vi "PSCOMMON_Toolbar Comond.vi"(7 "Pause？":bool, 8 "error in":errorcluster, 11 "Command":enum16{"Config", "Run", "Pause", "Stop", "Save"}(ring)) -> (0 "error out":errorcluster)   [LabVIEW 2016]
uses:
  X-Acquisition/DAQ Actor/API/PSDAQEG_Commoand Type.ctl
  Controls/Save Mode.ctl
  Ctrls/GlobeVaribles.vi
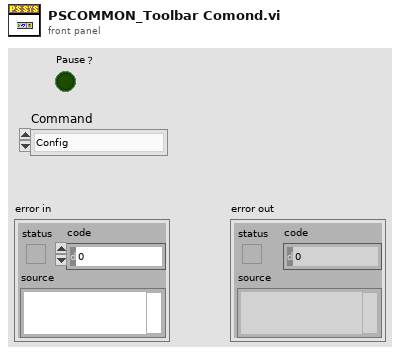
[diagram p1: front panel]
types:
  T1 = typedef "PSDAQEG_Commoand Type.ctl" = enum16{"Config", "Run", "Pause", "Stop", "Save"}
  T2 = enum16{"Run", "Pause", "Stop", "DAQ Chl", "Save", "Update Data", "Symbol Path", "DAQ DATA Queues", "None"}
  T3 = enum16{"Run", "Pause", "Stop", "DAQ Chl", "Save", "Update Data"}
  T4 = enum16{"open", "open or create", "create or replace", "create", "open (read-only)"}
  T5 = typedef "Global para Config.ctl" = cluster{"Timing":cluster{"SampleRate":i32}, "SavePara":cluster{"FlowDiskMode":T6, "SelectMode":T7, "FolderPath":path, "Filename":string, "FileNote":string, "AutoInterval":i32, "Template":path}, "ConfigDS Path*":path, "Tdms Ref*":refnum<k34>}
  T6 = typedef "File Save Mode.ctl" = i32
  T7 = typedef "Select Point Mode.ctl" = i32
  T8 = typedef "Save Mode.ctl" = i32
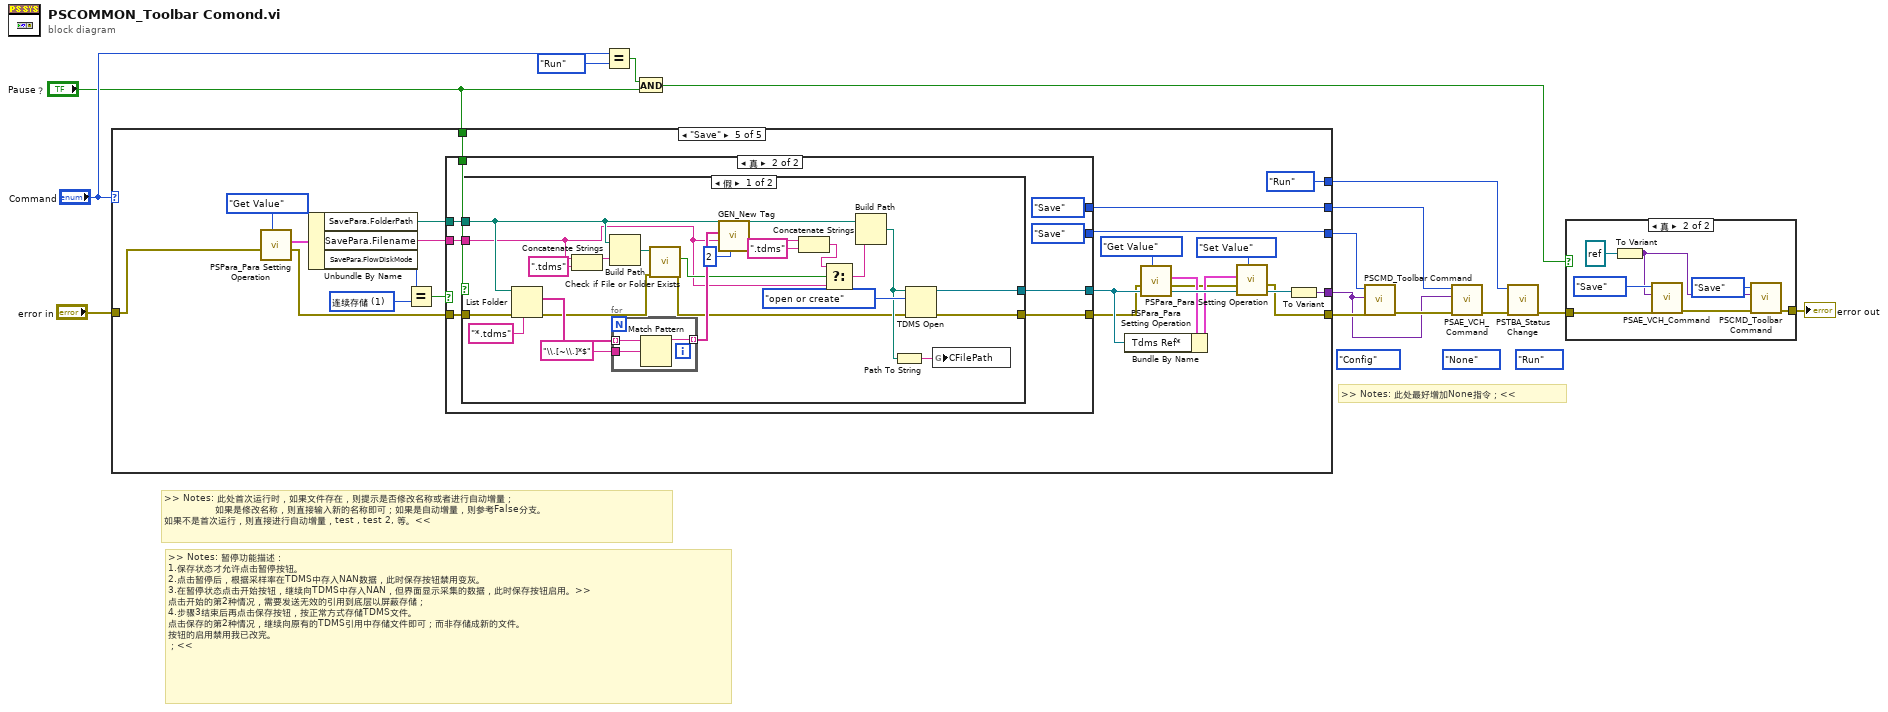
[diagram p0: block diagram]
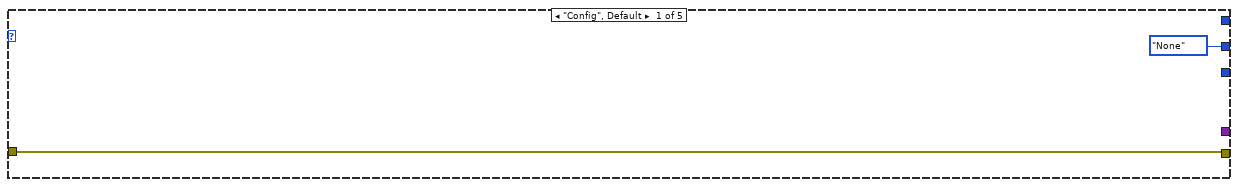
[diagram p3: hidden frame]
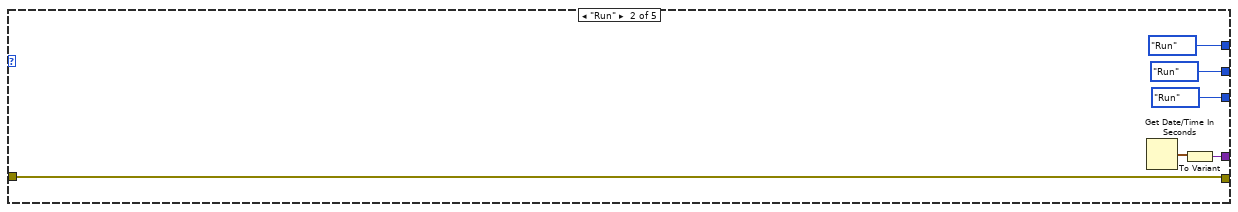
[diagram p4: hidden frame]
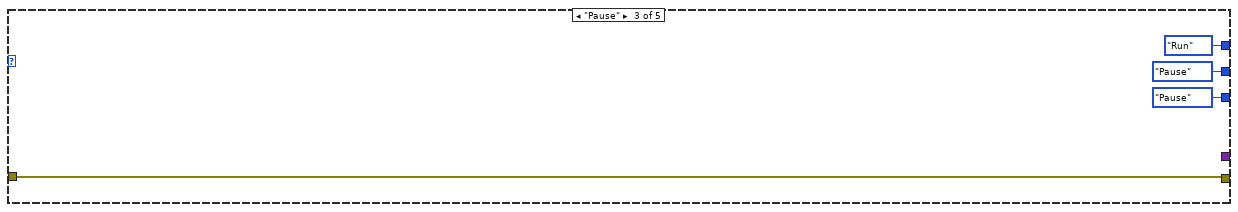
[diagram p5: hidden frame]
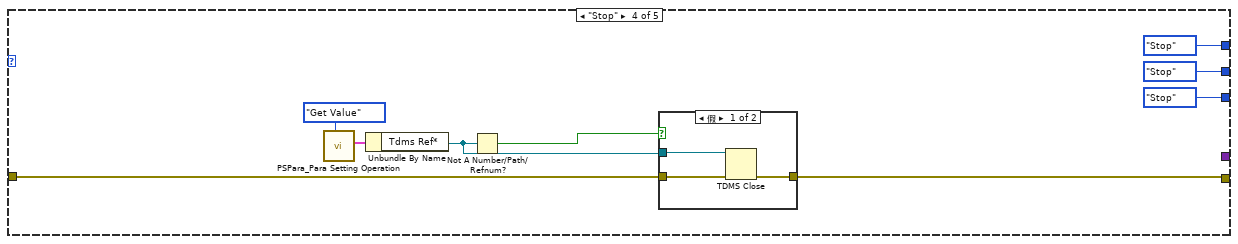
[diagram p6: hidden frame]
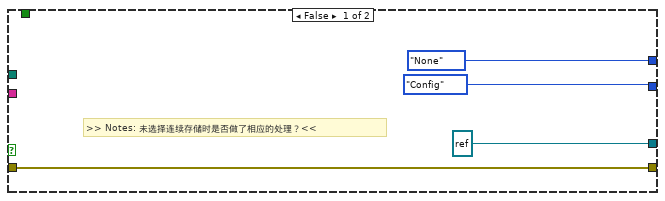
[diagram p8: hidden frame]
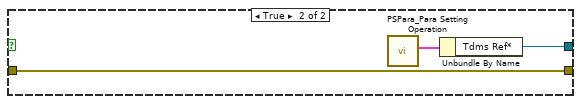
[diagram p9: hidden frame]
diagram:
  (unwired) enum16{"Run", "Stop"}."Run" ("Status")
  (unwired) PSDAQEG_Commoand_Type."Config" ("Command")
  (unwired) T2."None" ("Comd")
  # ">> Notes: 暂停功能描述：\n1.保存状态才允许点击暂停按钮。\n2.点击暂停后，根据采样率在TDMS中存入NAN数据，此时保存按钮禁用变灰。\n3.在暂停状态点击开始按钮，继续向TDMS中存入NAN，但界面显示采集的数据，此时保存按钮启用。>>\n点击开始的第2种情况，需要发送无效的引用到底层以屏蔽存储；\n4.步骤3结束后再点击保存按钮，按正常方式存储TDMS文件。\n点击保存的第2种情况，继续向原有的TDMS引用中存储文件即可；而非存储成新的文件。\n按钮的启用禁用我已改完。\n；<<"
  # ">> Notes: 此处最好增加None指令；<<"
  # ">> Notes: 此处首次运行时，如果文件存在，则提示是否修改名称或者进行自动增量；\n                 如果是修改名称，则直接输入新的名称即可；如果是自动增量，则参考False分支。\n如果不是首次运行，则直接进行自动增量，test , test 2, 等。<<"
  n1 = case shown="\"Save\"" "Command" {
    tunnel: [_ PSDAQEG_Commoand_Type."Run" ("Command") PSDAQEG_Commoand_Type."Pause" ("Command") PSDAQEG_Commoand_Type."Stop" ("Command") w58] -> w14
    tunnel: [T2."None" ("Comd") T2."Run" ("Comd") T2."Pause" ("Comd") T3."Stop" ("Comd") w57] -> w13
    tunnel: [_ enum16{"Run", "Stop"}."Run" ("Status") enum16{"Run", "Stop"}."Run" ("Status") enum16{"Run", "Stop"}."Stop" ("Status") enum16{"Run", "Stop"}."Run" ("Status")] -> w11
    tunnel: [_ w19 _ _ w60] -> w8
    tunnel: "error in" -> [w17 w22 w25 w32 w51]
    tunnel: [w17 w22 w25 w31 w59] -> w9
    tunnel: "Pause？" -> [_ _ _ _ w41]
    frame "Config", Default {
    }
    frame "Run" {
      n2 = Get Date/Time In Seconds() -> (seconds since 1Jan1904=w18:timestamp)
      n3 = To Variant(anything=w18) -> (Variant=w19:variant)
    }
    frame "Pause" {
    }
    frame "Stop" {
      n4 = call "PSPara_Para Setting Operation.vi"("Operation"=enum16{"Set Value", "Get Value", "Initialize"}."Get Value") -> ("_Para"=w33:T5)  [unwired: 9 in, 1 out]
      n5 = Unbundle By Name(w33) -> ("Tdms Ref*"=w29:refnum<k34>)
      n6 = Not A Number/Path/Refnum?(number/path/refnum=w29) -> (NaN/Path/Refnum?=w30:bool)
      n7 = case shown="假" w30 {
        tunnel: w32 -> [w39 w40]
        tunnel: [w38 w40] -> w31
        tunnel: w29 -> [w37 _]
        frame False {
          n8 = TDMS Close(8:w39, 11:w37) -> (0:w38:errorcluster)  [unwired: 1 out]
        }
        frame True {
        }
      }
    }
    frame "Save" {
      w49 = T8 1 items=["不存储", "连续存储"] ("y")
      n9 = call "PSPara_Para Setting Operation.vi"("Operation"=enum16{"Set Value", "Get Value", "Initialize"}."Get Value", "error in"=w51) -> ("error out"=w50:errorcluster, "_Para"=w56:T5)  [unwired: 8 in]
      n10 = Unbundle By Name(w56) -> ("SavePara.FolderPath"=w54:path, "SavePara.Filename"=w55:string, "SavePara.FlowDiskMode"=w53:T6)
      n11 = Equal?(x=w53, y=w49) -> (x = y?=w52:bool)
      n12 = case shown="真" w52 {
        tunnel: w55 -> [_ w69]
        tunnel: [w66 w74] -> w44
        tunnel: [refnum<k34> refnum ("tdms file out") w73] -> w61
        tunnel: w50 -> [w66 w72]
        tunnel: w54 -> [_ w70]
        tunnel: [PSDAQEG_Commoand_Type."Config" ("Command") PSDAQEG_Commoand_Type."Save" ("Command")] -> w58
        tunnel: [T2."None" ("Comd") T2."Save" ("Comd")] -> w57
        tunnel: w41 -> [_ w67]
        frame False {
          # ">> Notes: 未选择连续存储时是否做了相应的处理？<<"
        }
        frame True {
          n13 = case shown="假" w67 {
            tunnel: [w95 w103] -> w74
            tunnel: [w94 w101] -> w73
            tunnel: w72 -> [w93 w103]
            tunnel: w70 -> [w83 _]
            tunnel: w69 -> [w80 _]
            frame False {
              n14 = List Folder(path=w83, pattern="*.tdms", error in=w93) -> (filenames=w88:string[], error out=w76:errorcluster)  [unwired: 1 in, 2 out]
              n15 = Concatenate Strings(w80, ".tdms" ("字符串")) -> (w85:string)
              n16 = Build Path(base path=w83, name or relative path=w85) -> (appended path=w86:path)
              n17 = for {
                tunnel: "\\.[~\\.]*$" ("regular expression") -> [w100]
                tunnel: w88 -> [w99] mode=indexing
                tunnel: [w98] -> w87 mode=indexing
                n18 = Match Pattern(string=w99, regular expression=w100) -> (before substring=w98:string)  [unwired: 4 out]
              }
              n19 = call <vilib>:"Check if File or Folder Exists.vi"("error in (no error)"=w76, "path"=w86) -> ("error out"=w75:errorcluster, "file or folder exists?"=w82:bool)  [unwired: 7 in, 1 out]
              n20 = call "GEN_New Tag.vi"("Start Point"=2, "Basic"=w80, "Exist"=w87) -> ("Name"=w96:string)  [unwired: 7 in, 1 out]
              n21 = Concatenate Strings(w96, ".tdms" ("字符串")) -> (w81:string)
              n22 = Select(t=w81, s=w82, f=w80) -> (s? t:f=w79:string)
              n23 = Build Path(base path=w83, name or relative path=w79) -> (appended path=w78:path)
              n24 = Path To String(path=w78) -> (string=w77:string)
              n25 = TDMS Open(8:w75, 10:T4."open or create" ("operation (0:open)"), 11:w78) -> (0:w95:errorcluster, 3:w94:refnum<k34>)  [unwired: 4 in]
              n26 = global write "GlobeVaribles.vi" "CFilePath"(w77) -> ()
            }
            frame True {
              n27 = call "PSPara_Para Setting Operation.vi"() -> ("_Para"=w102:T5)  [unwired: 10 in, 1 out]
              n28 = Unbundle By Name(w102) -> ("Tdms Ref*"=w101:refnum<k34>)
            }
          }
        }
      }
      n29 = call "PSPara_Para Setting Operation.vi"("Operation"=enum16{"Set Value", "Get Value", "Initialize"}."Get Value", "error in"=w44) -> ("error out"=w43:errorcluster, "_Para"=w46:T5)  [unwired: 8 in]
      n30 = Bundle By Name(cluster=w46, "Tdms Ref*"=w61) -> (w45:T5)
      n31 = call "PSPara_Para Setting Operation.vi"("Operation"=enum16{"Set Value", "Get Value", "Initialize"}."Set Value", "error in"=w43, "_Para"=w45) -> ("error out"=w59:errorcluster)  [unwired: 7 in, 1 out]
      n32 = To Variant(anything=w61) -> (Variant=w60:variant)
    }
  }
  n33 = Equal?(x="Command", y=enum16{"Config", "Run", "Pause", "Stop", "Save"}."Run") -> (x = y?=w4:bool)
  n34 = And(x=w4, y="Pause？") -> (x .and. y?=w2:bool)
  n35 = call "PSCMD_Toolbar Command.vi"("error in"=w9, "Data"=w8, "Command"=w14) -> ("error out"=w15:errorcluster)  [unwired: 8 in]
  n36 = call "PSAE_VCH_Command.vi"("Error In (no error)"=w15, "Data"=w8, "Comd"=w13) -> ("Error Out"=w12:errorcluster)  [unwired: 8 in]
  n37 = call "PSTBA_Status Change.vi"("error in"=w12, "Status"=w11) -> ("error out"=w7:errorcluster)  [unwired: 9 in]
  n38 = case shown="真" w2 {
    tunnel: w7 -> [w104 w110]
    tunnel: [w104 w109] -> w6
    frame False {
    }
    frame True {
      n39 = To Variant(anything=refnum<k34> refnum ("tdms file out")) -> (Variant=w105:variant)
      n40 = call "PSAE_VCH_Command.vi"("Error In (no error)"=w110, "Data"=w105, "Comd"=T2."Save") -> ("Error Out"=w111:errorcluster)  [unwired: 8 in]
      n41 = call "PSCMD_Toolbar Command.vi"("error in"=w111, "Data"=w105, "Command"=PSDAQEG_Commoand_Type."Save") -> ("error out"=w109:errorcluster)  [unwired: 8 in]
    }
  }
  "error out" <- w6
